vi "Exp No 8 Application of Addition in Two Arrays Using LabView.vi"() -> ()   [LabVIEW 2010]
panel:
  out "Sum of First and Second Array":i32[](array[numeric])
  in  "Second Array":i32[](array[numeric])
  in  "First Array":i32[](array[numeric])
  in  "Number of Inputs":i32
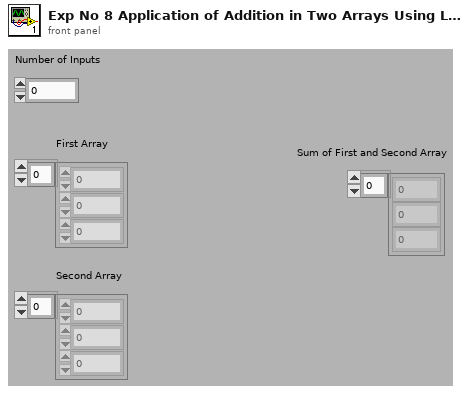
[diagram p1: front panel]
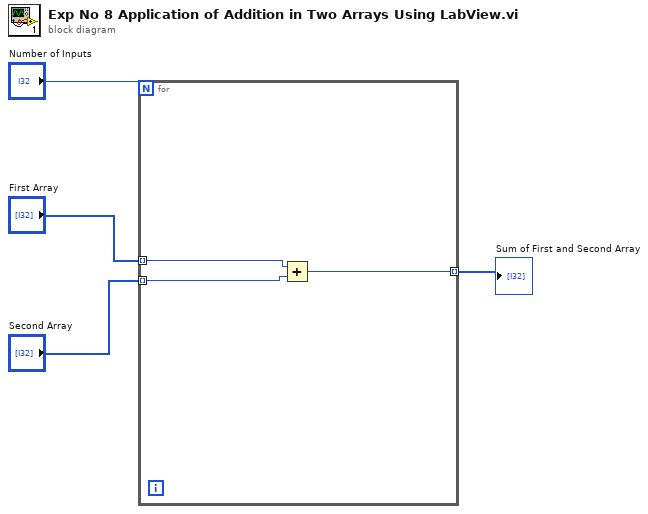
[diagram p0: block diagram]
diagram:
  n1 = for {
    N: "Number of Inputs" -> [_]
    tunnel: "Second Array" -> [w7] mode=indexing
    tunnel: "First Array" -> [w6] mode=indexing
    tunnel: [w5] -> w1 mode=indexing
    n2 = Add(x=w6, y=w7) -> (x+y=w5:i32)
  }
  "Sum of First and Second Array" <- w1
